vi "mod_CCDF accumulator.vi"(0 "IQ data (complex)":cluster{"t0":dbl, "dt":dbl, "Y":cdb[]} {"Y" format="%.2f"; "dt" format="%.2f"; "t0" format="%.2f"}, 1 "reset?":bool, 5 "upper limit":i32=10 format="%.0p", 7 "# bins":i32=500) -> (4 "CCDF":cluster{dbl[], dbl[]} {"?" format="%.2f"; "?" format="%.2f"}, 8 "overflow?":bool)   [LabVIEW 2020, in "niAMT.lvlib"]
uses:
  <vilib>/addons/Modulation/niAMT.lvlib
  <vilib>/Analysis/NI_AALPro.lvlib
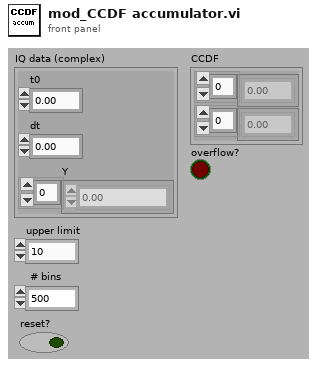
[diagram p1: front panel]
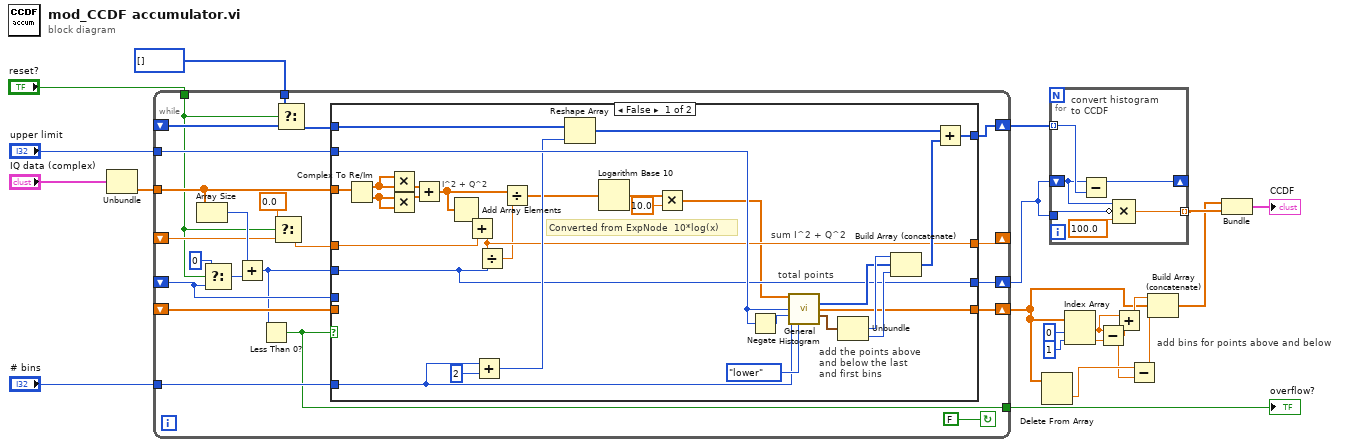
[diagram p0: block diagram]
diagram:
  # "add bins for points above and below"
  n1 = Unbundle("IQ data (complex)") -> ("Y"=w21:cdb[])  [unwired: 2 out]
  n2 = while {
    tunnel: w21 -> [w42]
    shift-right: [w27] -> w1
    shift-left: _ -> [w32]
    tunnel: "upper limit" -> [w41]
    shift-right: [w35] -> _
    shift-left: _ -> [w26]
    tunnel: "# bins" -> [w39]
    shift-right: [w40] -> w17
    shift-left: _ -> [w38]
    tunnel: i32[] [] -> [w36]
    tunnel: "reset?" -> [w24]
    tunnel: [w30] -> w3
    shift-right: [w29] -> w2
    shift-left: _ -> [w28]
    stop <- FALSE continue-if-true
    n3 = Array Size(array=w42) -> (size(s)=w34:i32)
    n4 = Select(t=0, s=w24, f=w32) -> (s? t:f=w33:i32)
    n5 = Add(x=w34, y=w33) -> (x+y=w22:i32)
    n6 = Less Than 0?(x=w22) -> (x < 0?=w30:bool)
    n7 = Select(t=0.0, s=w24, f=w26) -> (s? t:f=w25:dbl)
    n8 = Select(t=w36, s=w24, f=w38) -> (s? t:f=w37:i32[])
    n9 = case shown="False" w30 {
      tunnel: w42 -> [w69 _]
      tunnel: w41 -> [w67 _]
      tunnel: [w64 w76] -> w40
      tunnel: w39 -> [w62 _]
      tunnel: w37 -> [w57 w76]
      tunnel: w25 -> [w52 w75]
      tunnel: [w50 w75] -> w35
      tunnel: [w51 w77] -> w29
      tunnel: w28 -> [_ w77]
      tunnel: w32 -> [_ w74]
      tunnel: w22 -> [w49 _]
      tunnel: [w49 w74] -> w27
      frame False {
        # "Converted from ExpNode \t10*log(x)"
        # "total points"
        # "sum I^2 + Q^2"
        # "add the points above and below the last and first bins"
        # "I^2 + Q^2"
        n10 = Complex To Re/Im(x + iy=w69) -> (x=w73:dbl[], y=w70:dbl[])
        n11 = Multiply(x=w73, y=w73) -> (x*y=w71:dbl[])
        n12 = Multiply(x=w70, y=w70) -> (x*y=w72:dbl[])
        n13 = Add(x=w71, y=w72) -> (x+y=w54:dbl[])
        n14 = Add Array Elements(numeric array=w54) -> (sum=w53:dbl)
        n15 = Add(x=w53, y=w52) -> (x+y=w50:dbl)
        n16 = Add(x=w62, y=2) -> (x+y=w63:i32)
        n17 = Divide(x=w50, y=w49) -> (x/y=w48:dbl)
        n18 = Divide(x=w54, y=w48) -> (x/y=w45:dbl[])
        n19 = Reshape Array(w57, w63) -> (w65:i32[])
        n20 = Logarithm Base 10(1:w45) -> (0:w46:dbl[])
        n21 = Multiply(x=w46, y=10.0) -> (x*y=w44:dbl[])
        n22 = Negate(x=w67) -> (-x=w68:i32)
        n23 = call <vilib>:"General Histogram.vi"("X"=w44, "max"=w67, "min"=w68, "# bins"=w62, "inclusion"=enum32{"lower", "upper"}."lower") -> ("Histogram"=w56:i32[], "Axis"=w51:dbl[], "# outside"=w60:cluster{"total":i32, "below":i32, "above":i32})  [unwired: 1 in, 7 out]
        n24 = Unbundle(w60) -> ("below"=w59:i32, "above"=w58:i32)  [unwired: 1 out]
        n25 = Build Array (concatenate)(w59, w56, w58) -> (w55:i32[])
        n26 = Add(x=w65, y=w55) -> (x+y=w64:i32[])
      }
      frame True {
      }
    }
  }
  "overflow?" <- w3
  n27 = Delete From Array(array=w2) -> (deleted portion=w11:dbl)  [unwired: 2 in, 1 out]
  n28 = for {
    tunnel: w17 -> [w83] mode=indexing
    shift-right: [w79] -> _
    shift-left: w1 -> [w78]
    tunnel: w1 -> [w82]
    tunnel: [w80] -> w5 mode=indexing
    # "convert histogram to CCDF"
    n29 = Subtract(x=w78, y=w83) -> (x-y=w79:i32)
    n30 = Compound Arithmetic op=MULTIPLY(w78, invert w82, 100.0 ("value")) -> (w80:dbl)
  }
  n31 = Index Array(array=w2, index #1=0 ("index"), index #2=1 ("index")) -> (element #1=w14:dbl, element #2=w15:dbl)
  n32 = Subtract(x=w14, y=w15) -> (x-y=w10:dbl)
  n33 = Add(x=w14, y=w10) -> (x+y=w13:dbl)
  n34 = Subtract(x=w11, y=w10) -> (x-y=w9:dbl)
  n35 = Build Array (concatenate)(w13, w2, w9) -> (w4:dbl[])
  n36 = Bundle(w4, w5) -> (→"CCDF":cluster{dbl[], dbl[]})  [unwired: 1 out]
